vi "TabControlTypecast.vi"(0 "Ctl Refnum":refnum<vi>, 7 "Control Path In":string[](array[string]), 11 "Error In":errorcluster) -> (4 "Controls[]":refnum<vi>[](array[refnum]), 8 "Control Path Out":string[](array[string]), 15 "Error Out":errorcluster)   [LabVIEW 2016, in "Drona.lvlib" / "GetControlRef.lvlib"]
doc: "Gives the reference of controls present inside the tab control"
uses:
  GetControlRef.lvlib
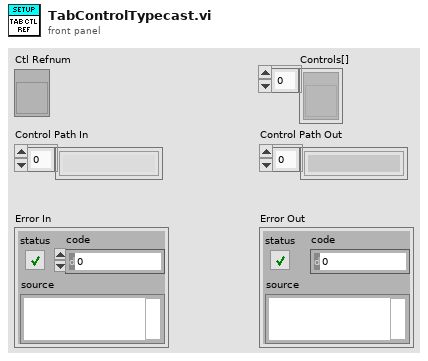
[diagram p1: front panel]
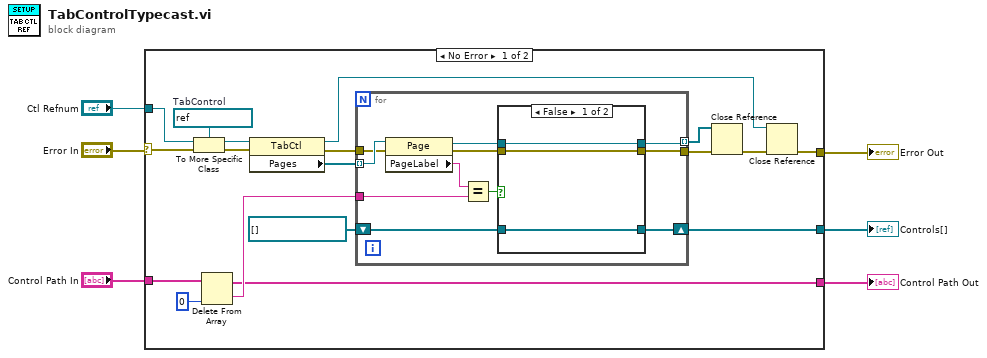
[diagram p0: block diagram]
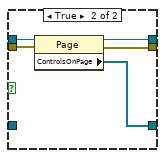
[diagram p2: hidden frame]
diagram:
  n1 = case shown="No Error" "Error In" {
    selector: "Error In" -> [w7 w45]
    tunnel: "Control Path In" -> [w24 w44]
    tunnel: "Ctl Refnum" -> [w23 _]
    tunnel: [w10 _] -> w4
    tunnel: [w9 w44] -> w3
    tunnel: [w8 w45] -> w2
    frame No Error {
      w20 = refnum<vi> refnum  # TabControl
      n2 = To More Specific Class(target class=w20, reference=w23, error in=w7) -> (specific class reference=w22:refnum<vi>, error out=w21:errorcluster)
      n3 = Delete From Array(array=w24, index=0) -> (deleted portion=w12:string, array with subset deleted=w9:string[])  [unwired: 1 in]
      n4 = property class="TabCtl"(reference=w22, error in=w21) -> (reference out=w14:refnum<vi>, error out=w17:errorcluster, "Pages"=w19:refnum<vi>[])
      n5 = for {
        tunnel: w19 -> [w35] mode=indexing
        tunnel: [w29] -> w18
        tunnel: w17 -> [w34]
        tunnel: [w26] -> w15 mode=indexing
        tunnel: w12 -> [w32]
        shift-right: [w27] -> w10
        shift-left: refnum<vi>[] [] ("ControlsOnPage") -> [w25]
        n6 = property class="Page"(reference=w35, error in=w34) -> (reference out=w28:refnum<vi>, error out=w30:errorcluster, "PageLabel"=w33:string)
        n7 = Equal?(x=w33, y=w32) -> (x = y?=w31:bool)
        n8 = case shown="False" w31 {
          tunnel: w30 -> [w38 w43]
          tunnel: [w38 w42] -> w29
          tunnel: w28 -> [w37 w41]
          tunnel: [w36 w40] -> w27
          tunnel: [w37 w39] -> w26
          tunnel: w25 -> [w36 _]
          frame False {
          }
          frame True {
            n9 = property class="Page"(reference=w41, error in=w43) -> (reference out=w39:refnum<vi>, error out=w42:errorcluster, "ControlsOnPage"=w40:refnum<vi>[])
          }
        }
      }
      n10 = Close Reference(reference=w15, error in (no error)=w18) -> (error out=w16:errorcluster)
      n11 = Close Reference(reference=w14, error in (no error)=w16) -> (error out=w8:errorcluster)
    }
    frame Error {
    }
  }
  "Controls[]" <- w4
  "Control Path Out" <- w3
  "Error Out" <- w2
